vi "close_data_file.vi"(8 "error in (no error)":errorcluster, 11 "Counter in":refnum<class "Counter.lvclass">) -> (0 "error out":errorcluster, 3 "Counter out":refnum<class "Counter.lvclass">)   [LabVIEW 2013, in "Counter.lvclass"]
uses:
  Counter.lvclass
  Counter.lvclass/Counter.ctl
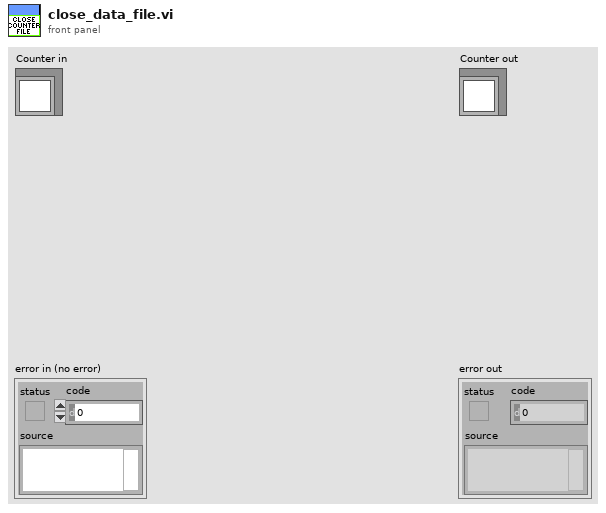
[diagram p1: front panel]
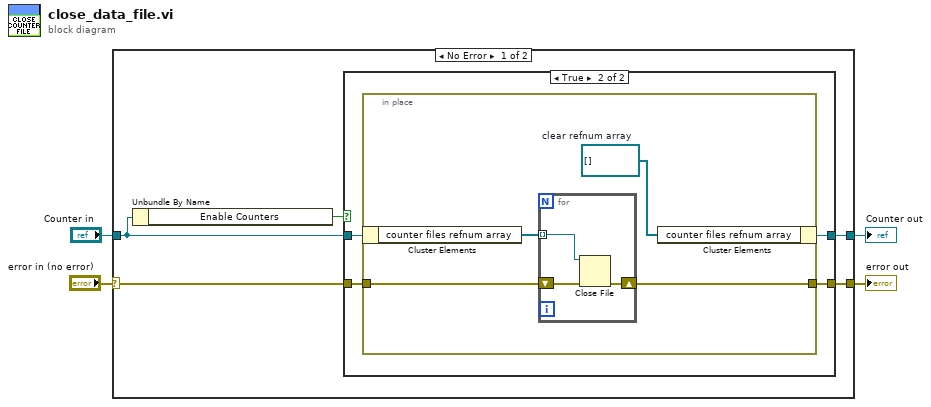
[diagram p0: block diagram]
diagram:
  n1 = case shown="No Error" "error in (no error)" {
    selector: "error in (no error)" -> [w9 w24]
    tunnel: [w8 w24] -> w3
    tunnel: [w7 w23] -> w1
    tunnel: "Counter in" -> [w6 w23]
    frame No Error {
      n2 = Unbundle By Name(w6) -> ("Enable Counters"=w5:bool)
      n3 = case shown="True" w5 {
        tunnel: w9 -> [w10 w15]
        tunnel: [w10 w14] -> w8
        tunnel: w6 -> [w11 w13]
        tunnel: [w11 w12] -> w7
        frame False {
        }
        frame True {
          n4 = in-place {
            in-place-border: w15 -> [w19]
            in-place-border: [w18] -> w14
            w16 = refnum<file>[] []  # clear refnum array
            n5 = in-place-cluster #1(w13) -> ("counter files refnum array"=w17:refnum<file>[])
            n6 = for {
              tunnel: w17 -> [w22] mode=indexing
              shift-right: [w20] -> w18
              shift-left: w19 -> [w21]
              n7 = Close File(refnum=w22, error in=w21) -> (error out=w20:errorcluster)  [unwired: 1 out]
            }
            n8 = in-place-cluster #1("counter files refnum array"=w16) -> (w12:refnum<class "Counter.lvclass">)
          }
        }
      }
    }
    frame Error {
    }
  }
  "error out" <- w3
  "Counter out" <- w1
